vi "ScanPressures.vi"() -> ()   [LabVIEW 2016]
uses:
  <userlib>/Fluigent/Fluigent MFCS/FluigentMFCS_Full.llb/MFCS_EZ Detect.vi
  <userlib>/Fluigent/Fluigent MFCS/FluigentMFCS_Full.llb/MFCS_EZ Initialization.vi
  <userlib>/Fluigent/Fluigent MFCS/FluigentMFCS_Full.llb/MFCS_EZ Read All Channels Pressure.vi
  <userlib>/Fluigent/Fluigent MFCS/FluigentMFCS_Full.llb/MFCS_EZ Write Channel Pressure.vi
panel:
  in  "Path":path
  out "dt":dbl[](array[numeric])
  out "All Channels Pressure":dbl[](array[numeric])
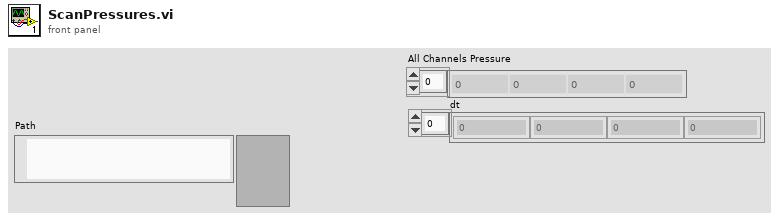
[diagram p1: front panel]
types:
  T1 = typedef "_EZmfcsSN.ctl" = u16
  T2 = typedef "_EZmfcsRefNum.ctl" = refnum<k1>
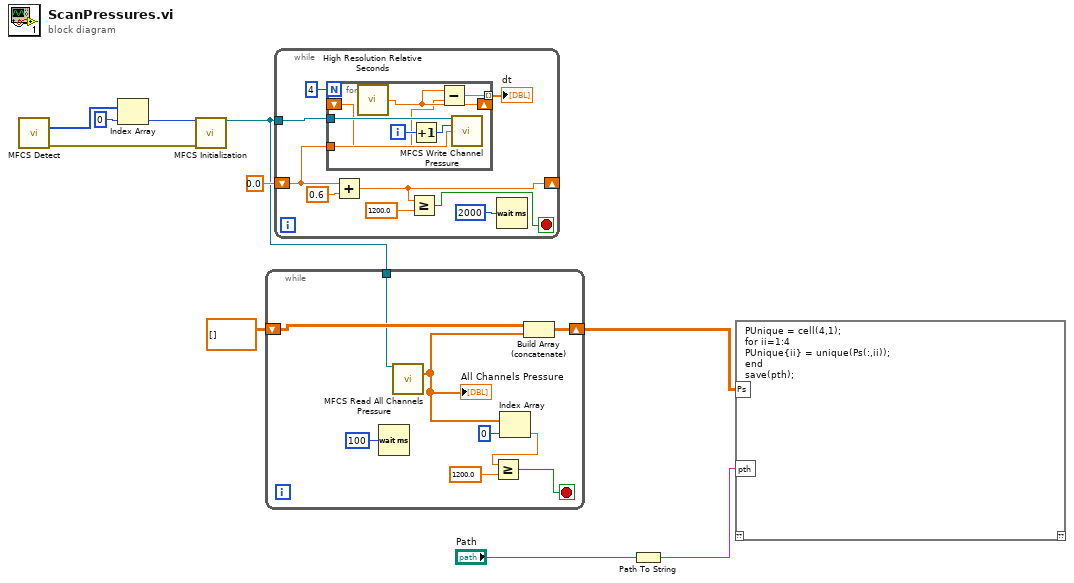
[diagram p0: block diagram]
diagram:
  n1 = call-poly <userlib>:"MFCS Detect.vi"() -> ("[SN MFCS_EZ]"=w10:T1[], "error out"=w7:errorcluster)  [unwired: 14 in]
  n2 = Index Array(array=w10, index=0) -> (element=w9:T1)
  n3 = call-poly <userlib>:"MFCS Initialization.vi"("SN MFCS_EZ"=w9, "error in (no error)"=w7) -> ("MFCS_EZ"=w5:T2)  [unwired: 11 in, 2 out]
  n4 = while {
    shift-right: [w19] -> w3
    shift-left: dbl[][] [] -> [w18]
    tunnel: w5 -> [w17]
    stop <- w12 stop-if-true
    n5 = Wait (ms)(milliseconds to wait=u32 100) -> ()  [unwired: 1 out]
    n6 = call-poly <userlib>:"MFCS Read All Channels Pressure.vi"("MFCS_EZ"=w17) -> ("All Channels Pressure"=w16:dbl[])  [unwired: 12 in, 2 out]
    "All Channels Pressure" <- w16
    n7 = Index Array(array=w16, index=0) -> (element=w13:dbl)
    n8 = Greater Or Equal?(x=w13, y=1200.0) -> (x >= y?=w12:bool)
    n9 = Build Array (concatenate)(w18, w16) -> (w19:dbl[][])
  }
  n10 = while {
    tunnel: w5 -> [w25]
    shift-right: [w23] -> _
    shift-left: 0.0 -> [w26]
    stop <- w24 stop-if-true
    n11 = for {
      N: 4 -> [_]
      tunnel: w26 -> [w35]
      tunnel: w25 -> [w32]
      shift-right: [w31] -> _
      shift-left: _ -> [w30]
      tunnel: [w29] -> w20 mode=indexing
      i -> [w34]
      n12 = call <vilib>:"High Resolution Relative Seconds.vi"() -> ("relative seconds"=w31:dbl)
      n13 = Increment(x=w34) -> (x+1=w33:i32)
      n14 = Subtract(x=w31, y=w30) -> (x-y=w29:dbl)
      n15 = call-poly <userlib>:"MFCS Write Channel Pressure.vi"("MFCS_EZ"=w32, "Channel Number (default=1)"=w33, "Pressure (mBar)"=w35) -> ()  [unwired: 11 in, 2 out]
    }
    "dt" <- w20
    n16 = Add(x=w26, y=0.6) -> (x+y=w23:dbl)
    n17 = Greater Or Equal?(x=w23, y=1200.0) -> (x >= y?=w24:bool)
    n18 = Wait (ms)(milliseconds to wait=u32 2000) -> ()  [unwired: 1 out]
  }
  n19 = Path To String(path="Path") -> (string=w1:string)
  n20 = script code="PUnique = cell(4,1);\nfor ii=1:4\nPUnique{ii} = unique(Ps(:,ii));\nend\nsave(pth);"("Ps"=w3, "pth"=w1) -> ()  [unwired: 1 in, 1 out]
